vi "Bin Pixels 8x8 (SubVI).vi"(5 "Threshold":u8=32, 7 "Image Width":u16=3072, 8 "Input Valid":bool, 11 "Data In":u64) -> (0 "Output Valid":bool, 3 "Pixel Data":bool)   [LabVIEW 2015]
uses:
  <vilib>/rvi/DataTransferAndStorage/Container/Common/niFpgaContainerGetUniqueNameForEmu.vi
  <vilib>/rvi/DataTransferAndStorage/Container/Common/niFpgaContainerSetEmuInfo.vi
  <vilib>/rvi/eio/common/nirviEmuReportErrorAndStop.vi
  <vilib>/rvi/Emulation/niFpgaEmulationIsFPGAContextNoSignature.vi
  <vilib>/rvi/Emulation/niFpgaSctlEmulationGetInTimedLoop.vi
  <vilib>/rvi/errors/niFpgaSetErrorForExecOnDevCompSimple.vi
  <vilib>/rvi/FIFO/Fifo_Resource/nirvififoEmulationSetSize.vi
  <vilib>/rvi/FIFO/Fifo_Resource/nirviFifoEmulationQueueMgr.vi
  <instcachedir>/0/nirviFifoEmulationQueueMgr_E5CAEC123FF24DC58D834DCA3CDAA9B5.lvgen/nirviFifoEmulationQueueMgr_E5CAEC123FF24DC58D834DCA3CDAA9B5_001.vi
  <vilib>/Utility/error.llb/Clear Errors.vi
  <vilib>/rvi/FIFO/Fifo_Resource/nirvififoEmulationCreateLock.vi
  <vilib>/rvi/Emulation/niFpgaProcessEmulError.vi
  <vilib>/rvi/FIFO/Fifo_Resource/nirvififoEmulationObtainLock.vi
  <vilib>/rvi/FIFO/Fifo_Resource/nirvififoEmulationReleaseLock.vi
  <vilib>/rvi/occurrence/nirviWaitOnOccurrenceBase.vi
  <vilib>/rvi/errors/nirviReportUnexpectedCaseInternalError.vi
  <vilib>/rvi/errors/nirviReportUnexpectedCaseInternalError (U32).vi
  <vilib>/rvi/FIFO/Fifo_Resource/nirvififoEmulationDetermineInputValidOut.vi
  <vilib>/rvi/LocalResourceManager/LocalResourceManager.xnode
  <vilib>/rvi/DataTransferAndStorage/Container/XNode/niFpgaContainer.xnode
  <vilib>/rvi/FIFO/Fifo_Resource/nirvififoEmulationRead.vi
  <vilib>/rvi/FIFO/Fifo_Resource/nirvififoEmulationWrite.vi
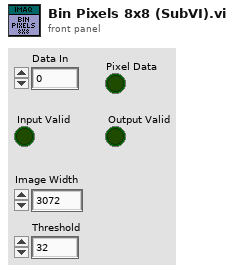
[diagram p1: front panel]
types:
  T1 = cluster{"Numeric Control":u8, "Numeric Control":u8, "Numeric Control":u8, "Numeric Control":u8, "Numeric Control":u8, "Numeric Control":u8, "Numeric Control":u8, "Numeric Control":u8}
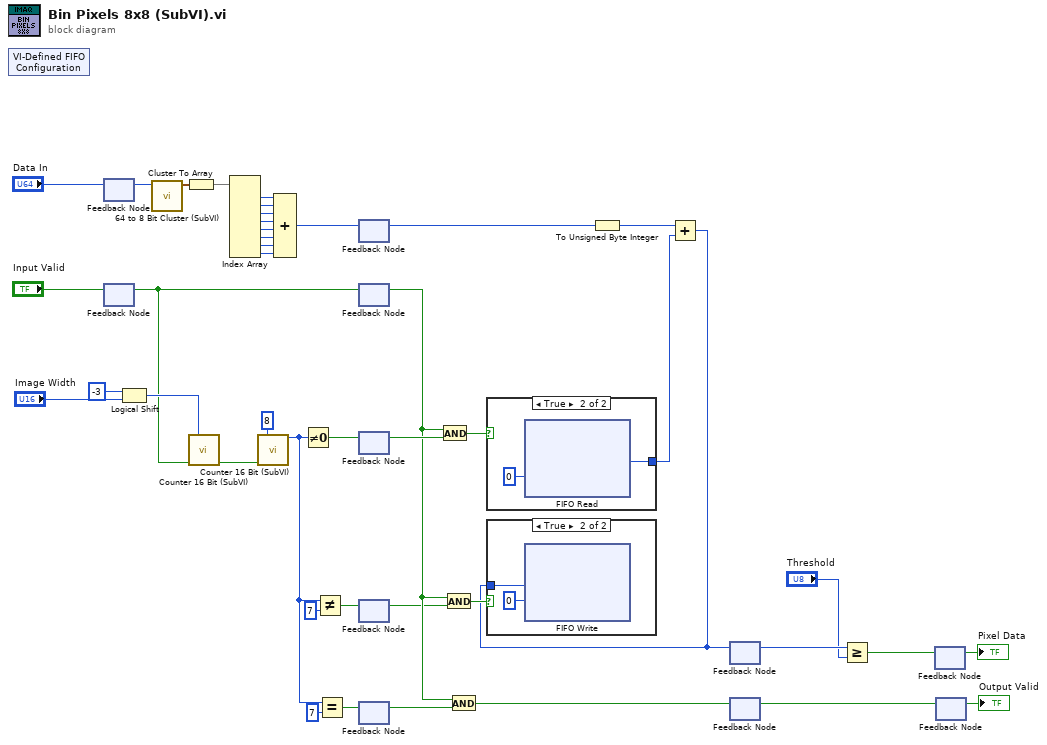
[diagram p0: block diagram]
diagram:
  n1 = xnode "VI-Defined FIFO Configuration"() -> ()  [unwired: 1 out]
  n2 = feedback #1() -> (w42:u64)  [unwired: 1 in]
  n3 = feedback-in #1("Data In") -> ()
  n4 = feedback-in #2("Input Valid") -> ()
  n5 = feedback #2() -> (w22:bool)  [unwired: 1 in]
  n6 = Logical Shift(y=i16 -3, x="Image Width") -> (x << y=w24:u16)
  n7 = call "64 to 8 Bit Cluster (SubVI).vi"("Data In"=w42) -> ("Data Out"=w40:T1)  [unwired: 10 in]
  n8 = Cluster To Array(cluster=w40) -> (array=w39:u8[])
  n9 = call "Counter 16 Bit (SubVI).vi"("Max. Count"=w24, "Enable"=w22) -> ("Count End?"=w26:bool)  [unwired: 11 in, 2 out]
  n10 = Index Array(array=w39) -> (element #1=w38:u8, element #2=w37:u8, element #3=w36:u8, element #4=w35:u8, element #5=w33:u8, element #6=w32:u8, element #7=w31:u8, element #8=w30:u8)  [unwired: 8 in]
  n11 = call "Counter 16 Bit (SubVI).vi"("Max. Count"=u16 8, "Enable"=w26) -> ("Count"=w7:u16)  [unwired: 11 in, 2 out]
  n12 = Compound Arithmetic op=ADD(w38, w37, w36, w35, w33, w32, w31, w30) -> (w29:u8)
  n13 = Not Equal To 0?(x=w7) -> (x != 0?=w20:bool)
  n14 = Not Equal?(x=w7, y=u16 7) -> (x != y?=w16:bool)
  n15 = Equal?(x=w7, y=u16 7) -> (x = y?=w5:bool)
  n16 = feedback-in #3(w29) -> ()
  n17 = feedback #3() -> (w14:u8)  [unwired: 1 in]
  n18 = feedback-in #4(w22) -> ()
  n19 = feedback #4() -> (w10:bool)  [unwired: 1 in]
  n20 = feedback #5() -> (w19:bool)  [unwired: 1 in]
  n21 = feedback-in #5(w20) -> ()
  n22 = feedback #6() -> (w9:bool)  [unwired: 1 in]
  n23 = feedback-in #6(w16) -> ()
  n24 = feedback-in #7(w5) -> ()
  n25 = feedback #7() -> (w3:bool)  [unwired: 1 in]
  n26 = And(x=w10, y=w19) -> (x .and. y?=w18:bool)
  n27 = And(x=w10, y=w9) -> (x .and. y?=w15:bool)
  n28 = And(x=w10, y=w3) -> (x .and. y?=w8:bool)
  n29 = case shown="True" w18 {
    tunnel: [_ w44] -> w13
    frame False {
    }
    frame True {
      n30 = xnode ("FIFO Read")("Timeout"=0) -> ("Element"=w44:u8)  [unwired: 1 in, 2 out]
    }
  }
  n31 = To Unsigned Byte Integer(number=w14) -> (unsigned 8bit integer=w2:u8)
  n32 = Add(x=w2, y=w13) -> (x+y=w12:u8)
  n33 = case shown="True" w15 {
    tunnel: w12 -> [_ w46]
    frame False {
    }
    frame True {
      n34 = xnode ("FIFO Write")("Element"=w46, "Timeout"=0) -> ()  [unwired: 1 in, 2 out]
    }
  }
  n35 = feedback #8() -> (w11:u8)  [unwired: 1 in]
  n36 = feedback-in #8(w12) -> ()
  n37 = feedback-in #9(w8) -> ()
  n38 = feedback #9() -> (w4:bool)  [unwired: 1 in]
  n39 = Greater Or Equal?(x=w11, y="Threshold") -> (x >= y?=w28:bool)
  n40 = feedback #10() -> (→"Pixel Data":bool)  [unwired: 1 in]
  n41 = feedback-in #10(w28) -> ()
  n42 = feedback #11() -> (→"Output Valid":bool)  [unwired: 1 in]
  n43 = feedback-in #11(w4) -> ()
